vi "Create Notifiers.vi"(8 "error in":errorcluster) -> (0 "error out":errorcluster, 3 "output cluster":T1)   [LabVIEW 2015]
uses:
  Notifiers.ctl
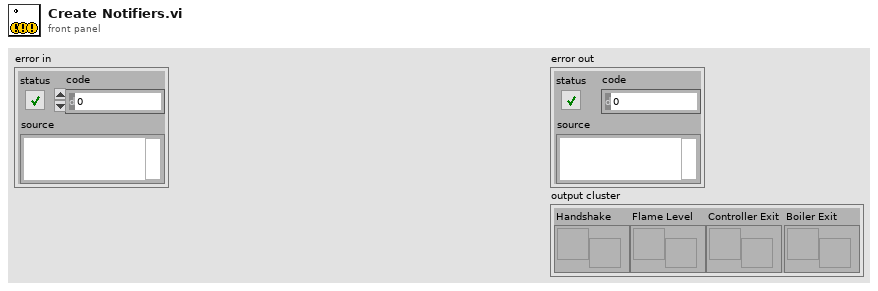
[diagram p1: front panel]
types:
  T1 = typedef "Notifiers.ctl" = cluster{"Handshake":refnum<notifier>, "Flame Level":refnum<notifier>, "Controller Exit":refnum<notifier>, "Boiler Exit":refnum<notifier>}
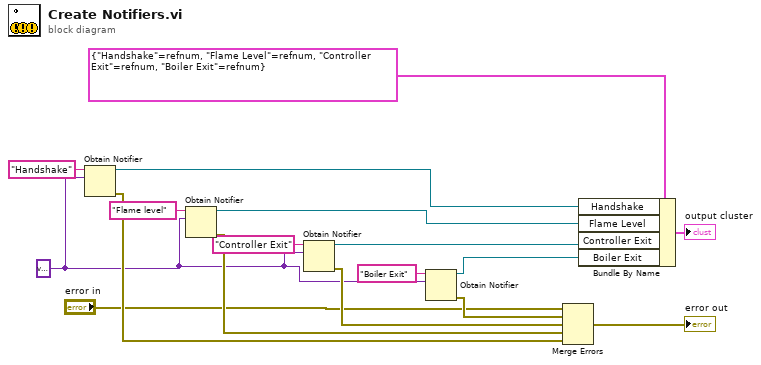
[diagram p0: block diagram]
diagram:
  w11 = variant ("element data type")
  n1 = Obtain Notifier(name (unnamed)="Handshake", notification data type=w11) -> (notifier out=w3:refnum<notifier>, error out=w14:errorcluster)  [unwired: 2 in, 1 out]
  n2 = Obtain Notifier(name (unnamed)="Flame level", notification data type=w11) -> (notifier out=w6:refnum<notifier>, error out=w15:errorcluster)  [unwired: 2 in, 1 out]
  n3 = Obtain Notifier(name (unnamed)="Controller Exit", notification data type=w11) -> (notifier out=w5:refnum<notifier>, error out=w16:errorcluster)  [unwired: 2 in, 1 out]
  n4 = Obtain Notifier(name (unnamed)="Boiler Exit", notification data type=w11) -> (notifier out=w4:refnum<notifier>, error out=w17:errorcluster)  [unwired: 2 in, 1 out]
  n5 = Merge Errors("error in", w17, w16, w15, w14) -> (→"error out":errorcluster)
  n6 = Bundle By Name(cluster=T1 {"Handshake"=refnum, "Flame Level"=refnum, "Controller Exit"=refnum, "Boiler Exit"=refnum}, "Handshake"=w3, "Flame Level"=w6, "Controller Exit"=w5, "Boiler Exit"=w4) -> (→"output cluster":T1)
